vi "Get Bucket RequestPayment Configuration.vi"(4 "Region":T1, 8 "error in (no error)":errorcluster, 9 "Bucket":string) -> (0 "error out":errorcluster, 3 "RequestPaymentConfiguration":T2)   [LabVIEW 2015, in "LV Interface for Amazon S3.lvlib"]
doc: "This operation <B>returns the request payment configuration</B> of a bucket. To use this version of the operation, <B>you must be the bucket owner</B>."
uses:
  LV Interface for Amazon S3.lvlib
  Typedefs/AMZ_S3_API_RequestPaymentConfig.ctl
  Typedefs/AMZ_S3_Payer.ctl
  Typedefs/AMZ_S3_LocationConstraint.ctl
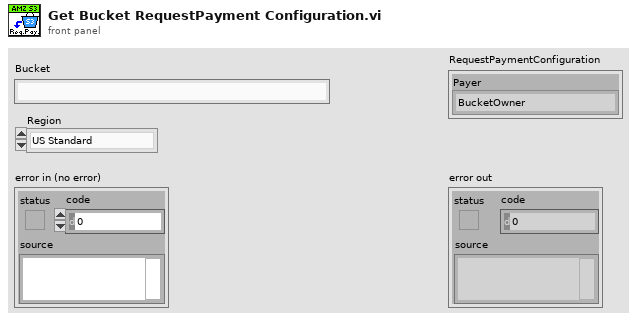
[diagram p1: front panel]
types:
  T1 = typedef "LV Interface for Amazon S3.lvlib/AMZ_S3_LocationConstraint.ctl" = enum16{"US Standard", "us-east-2", "us-west-1", "us-west-2", "ap-northeast-1", "ap-northeast-2", "ap-southeast-1", "ap-southeast-2", "ca-central-1", "eu-central-1", "eu-west-1", "eu-west-2", "sa-east-1"}
  T2 = typedef "LV Interface for Amazon S3.lvlib/AMZ_S3_API_RequestPaymentConfig.ctl" = cluster{"Payer":T3}
  T3 = typedef "LV Interface for Amazon S3.lvlib/AMZ_S3_Payer.ctl" = enum16{"BucketOwner", "Requester"}
  T4 = typedef "LV Interface for Amazon S3.lvlib/AMZ_S3_Call Results.ctl" = enum16{"Success", "UndefinedError", "AccessDenied", "AccountProblem", "AmbiguousGrantByEmailAddress", "BadDigest", "BucketAlreadyExists", "BucketAlreadyOwnedByYou", "BucketNotEmpty", "CredentialsNotSupported", "CrossLocationLoggingProhibited", "EntityTooSmall", "EntityTooLarge", "ExpiredToken", "IllegalVersioningConfigurationException", "IncompleteBody", "IncorrectNumberOfFilesInPostRequest", "InlineDataTooLarge", "InternalError", "InvalidAccessKeyId", "InvalidAddressingHeader", "InvalidArgument", "InvalidBucketName", "InvalidDigest", "InvalidLocationConstraint", "InvalidPart", "InvalidPartOrder", "InvalidPayer", "InvalidPolicyDocument", "InvalidRange", "InvalidSecurity", "InvalidSOAPRequest", "InvalidStorageClass", "InvalidTargetBucketForLogging", "InvalidToken", "InvalidURI", "KeyTooLong", "MalformedACLError", "MalformedPOSTRequest", "MalformedXML", "MaxMessageLengthExceeded", "MaxPostPreDataLengthExceededError", "MetadataTooLarge", "MethodNotAllowed", "MissingAttachment", "MissingContentLength", "MissingRequestBodyError", "MissingSecurityElement", "MissingSecurityHeader", "NoLoggingStatusForKey", "NoSuchBucket", "NoSuchKey", "NoSuchUpload", "NoSuchVersion", "NotImplemented", "NotSignedUp", "OperationAborted", "PermanentRedirect", "PreconditionFailed", "Redirect", "RequestIsNotMultiPartContent", "RequestTimeout", "RequestTimeTooSkewed", "RequestTorrentOfBucketError", "SignatureDoesNotMatch", "SlowDown", "TemporaryRedirect", "TokenRefreshRequired", "TooManyBuckets", "UnexpectedContent", "UnresolvableGrantByEmailAddress", "UserKeyMustBeSpecified", "LabVIEWError"}
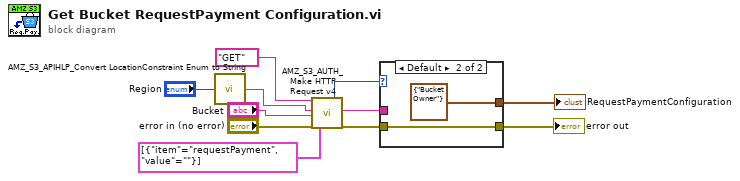
[diagram p0: block diagram]
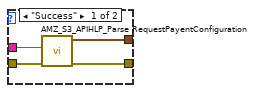
[diagram p2: hidden frame]
diagram:
  n1 = call "AMZ_S3_APIHLP_Convert LocationConstraint Enum to String.vi"("Location"="Region") -> ("Location String"=w2:string)  [unwired: 4 in]
  n2 = call "AMZ_S3_AUTH_Make HTTP Request v4.vi"("HTTP-Verb"="GET", "Region"=w2, "Bucket"="Bucket", "error in"="error in (no error)", "request parameters"=cluster{"item":string, "value":string}[] [{"item"="requestPayment", "value"=""}]) -> ("Call Result"=w7:T4, "response body"=w8:string, "error out"=w9:errorcluster)  [unwired: 11 in, 1 out]
  n3 = case shown="Default" w7 {
    tunnel: w9 -> [w15 w16]
    tunnel: w8 -> [w14 _]
    tunnel: [w13 w16] -> w11
    tunnel: [w12 T2 {"Payer"=enum."BucketOwner"} ("RequestPaymentConfiguration")] -> w10
    frame "Success" {
      n4 = call "AMZ_S3_APIHLP_Parse RequestPayentConfiguration.vi"("error in (no error)"=w15, "Response body"=w14) -> ("error out"=w13:errorcluster, "RequestPaymentConfiguration"=w12:T2)  [unwired: 8 in]
    }
    frame Default {
    }
  }
  "error out" <- w11
  "RequestPaymentConfiguration" <- w10
